vi "Connect.vi"(8 "error in":errorcluster, 11 "DB-SQLite in":refnum<class "DB-SQLite.lvclass">) -> (0 "error out":errorcluster, 3 "DB-SQLite out":refnum<class "DB-SQLite.lvclass">)   [LabVIEW 2020, in "hse-db-sqlite.lvlib" / "DB-SQLite.lvclass"]
doc: "____\nHAMPEL SOFTWARE ENGINEERING v1.4.0 (2023-12-19 09:52)"
uses:
  DB-SQLite.lvclass
  DB-SQLite.lvclass/DB-SQLite.ctl
  <vilib>/drjdpowell/SQLite Library/SQL Connection/Open (string).vi
  <vilib>/drjdpowell/SQLite Library/SQL Connection/Connection.lvclass
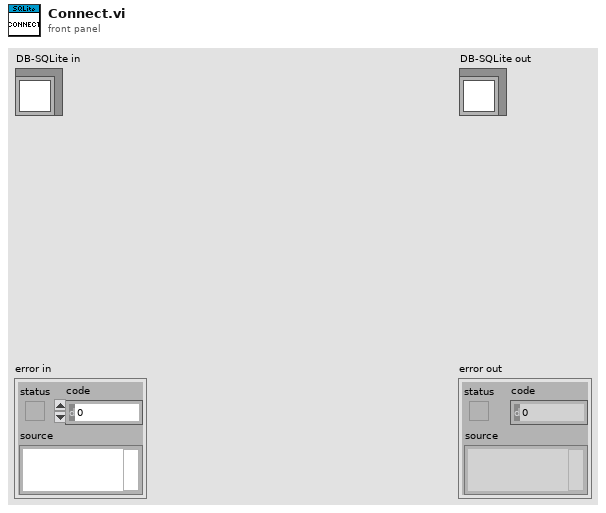
[diagram p1: front panel]
types:
  T1 = enum16{"New or existing", "Existing", "Read only"}
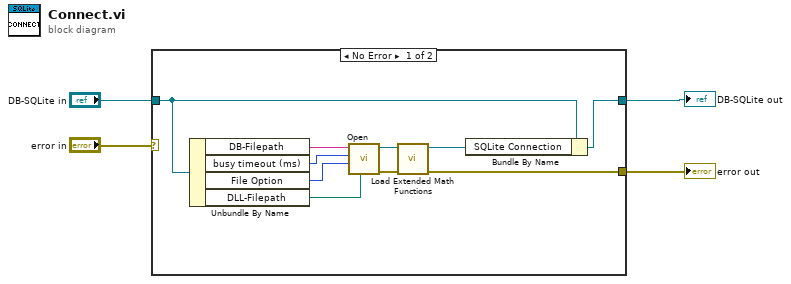
[diagram p0: block diagram]
diagram:
  n1 = case shown="No Error" "error in" {
    selector: "error in" -> [_ w16]
    tunnel: [w6 w16] -> w3
    tunnel: "DB-SQLite in" -> [w14 w15]
    tunnel: [w13 w15] -> w1
    frame No Error {
      n2 = Unbundle By Name(w14) -> ("DB-Filepath"=w10:string, "busy timeout (ms)"=w9:i32, "File Option"=w8:T1, "DLL-Filepath"=w5:path)
      n3 = call-poly <vilib>:"Open.vi"("SQLite Library Path"=w5, "File Option"=w8, "busy timeout (ms)"=w9, "db file"=w10) -> ("error out"=w12:errorcluster, "SQLite Connection"=w11:refnum<class "Connection.lvclass">)  [unwired: 6 in]
      n4 = call <vilib>:"Load Extended Math Functions.vi"("error in (no error)"=w12, "SQLite Connection in"=w11) -> ("error out"=w6:errorcluster, "SQLite Connection"=w7:refnum<class "Connection.lvclass">)  [unwired: 8 in]
      n5 = Bundle By Name(cluster=w14, "SQLite Connection"=w7) -> (w13:refnum<class "DB-SQLite.lvclass">)
    }
    frame Error {
    }
  }
  "error out" <- w3
  "DB-SQLite out" <- w1
